vi "EnFlo_Lab_Temp_Control.vi"(0 "Current Time":dbl) -> ()   [LabVIEW 2016]
uses:
  <vilib>/Analysis/NI_AALPro.lvlib
panel:
  out "Integral Term":dbl
  out "Derivative Term":dbl
  out "Proportional Term":dbl
  out "Cooling from Tunnel Exit Duct kW":dbl
  out "Exit Heater Dem Power %":dbl
  in  "Ki":dbl=0.025 format="%.3f"
  in  "Kp":dbl=30.0 format="%.2f"
  in  "Kd":dbl=50.0 format="%.2f"
  in  "Derivative History":i32=20
  out "EnFlo_Tunnel:Temp:Pre_Inlet_Average":dbl
  out "EnFlo_Tunnel:Exit Duct:Dem Temp":dbl
  out "Reduction in air temp from ambient":dbl
  out "Heat Extraction Value in kW":dbl
  out "EnFlo Lab:Desired:Air Temp":dbl
  out "Temperature Error":dbl
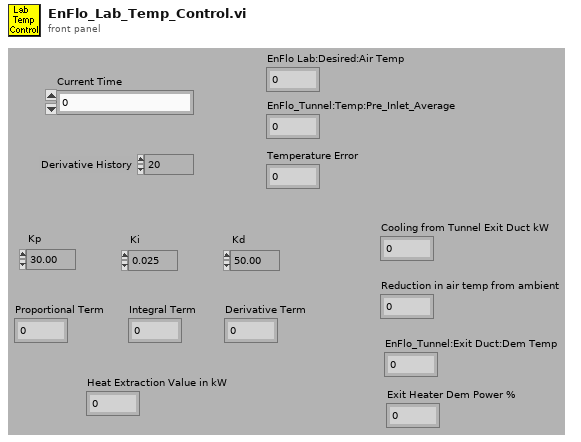
[diagram p1: front panel]
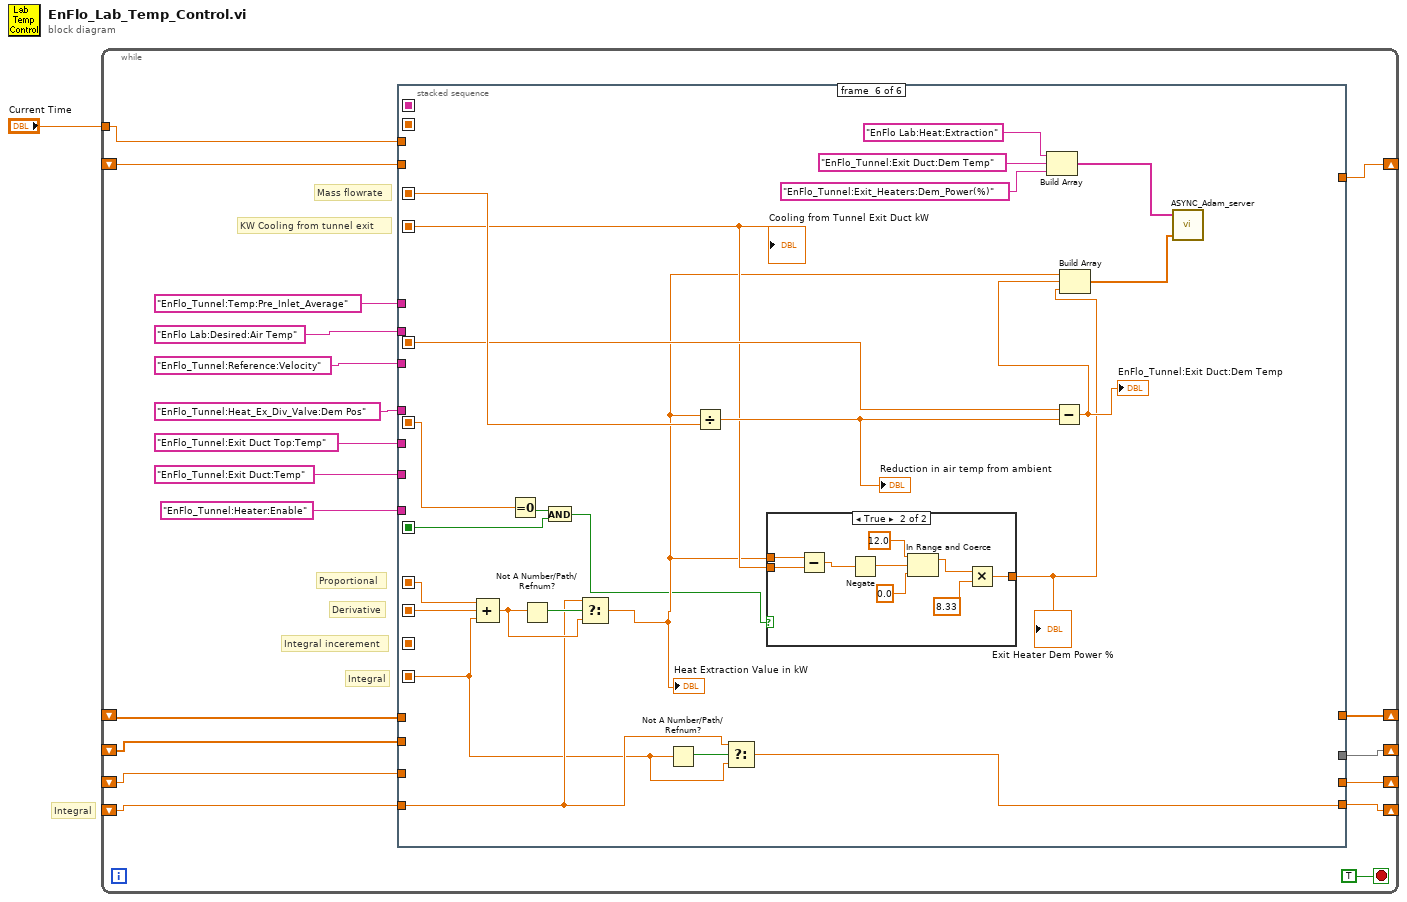
[diagram p0: block diagram]
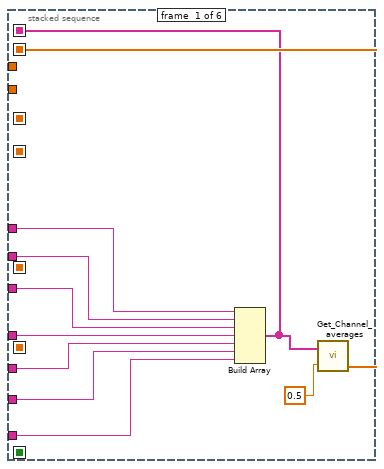
[diagram p2: hidden frame]
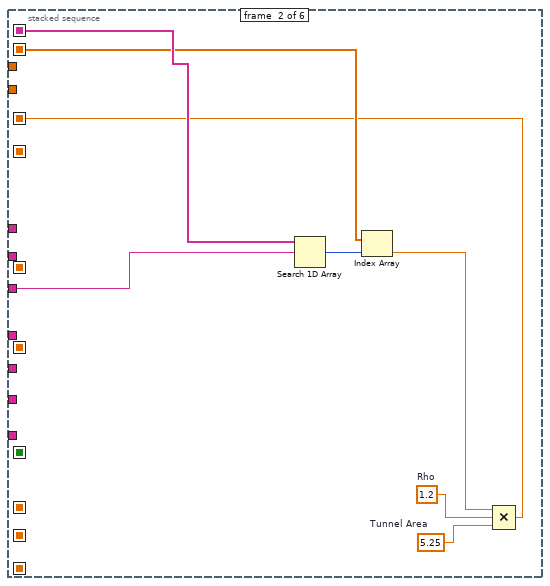
[diagram p3: hidden frame]
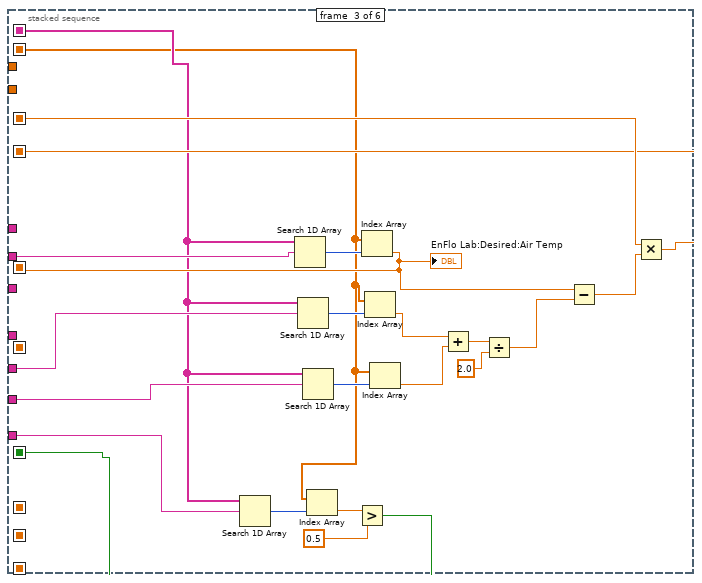
[diagram p4: hidden frame]
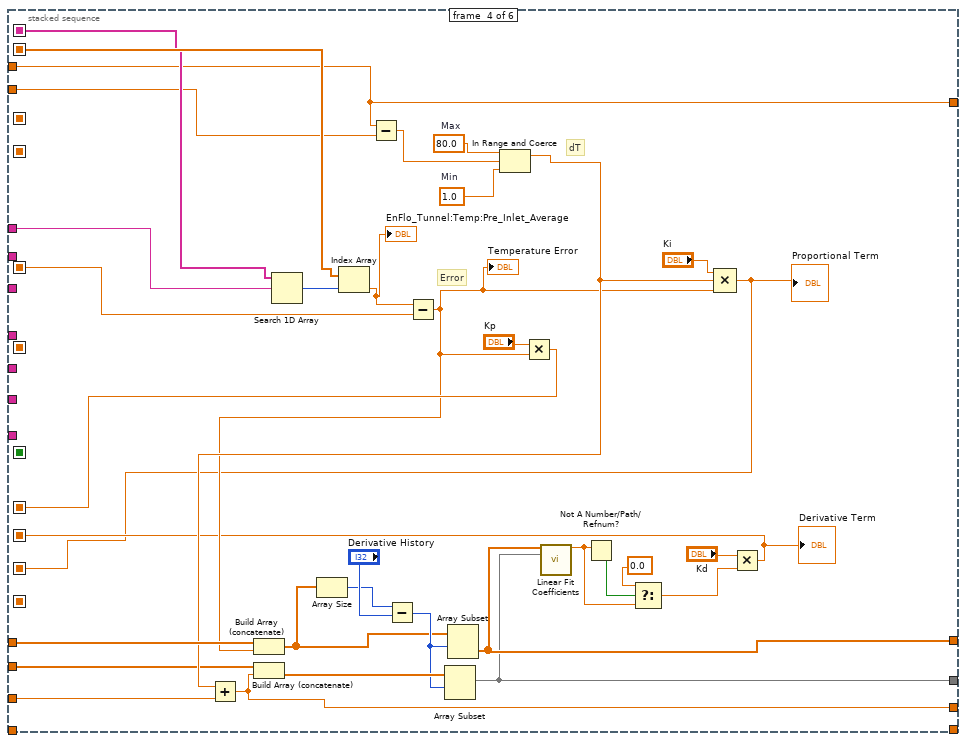
[diagram p5: hidden frame]
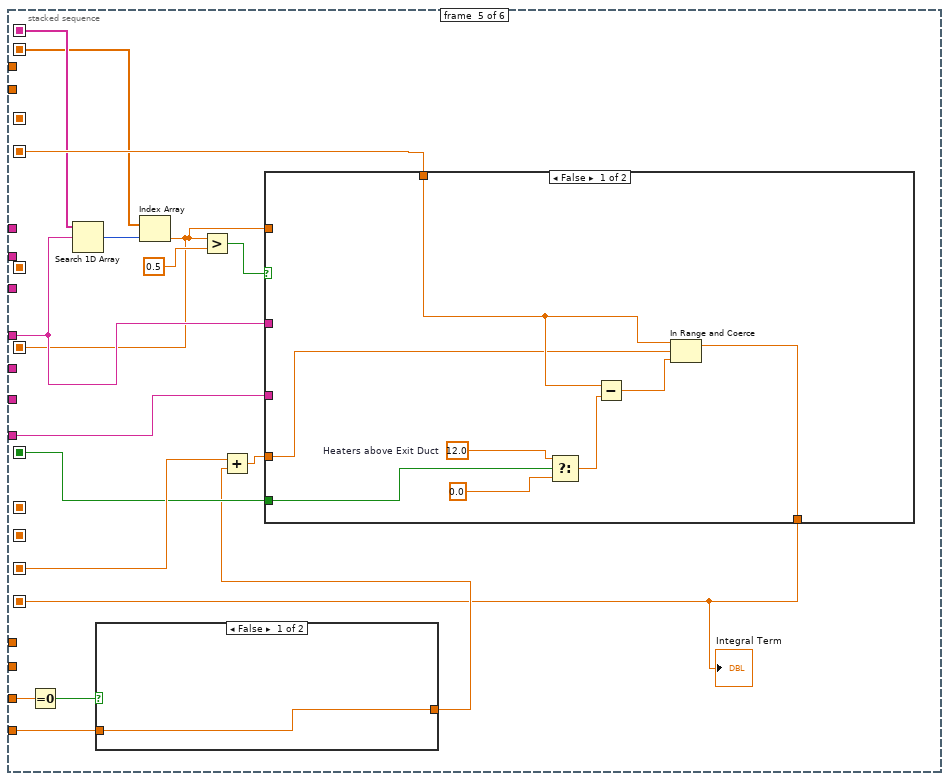
[diagram p6: hidden frame]
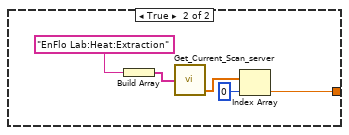
[diagram p7: hidden frame]
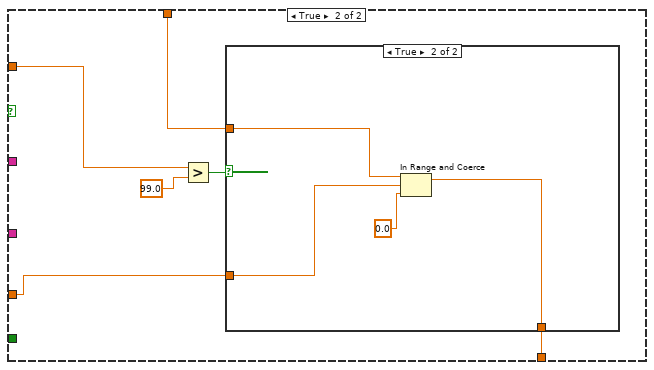
[diagram p8: hidden frame]
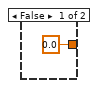
[diagram p10: hidden frame]
diagram:
  # "Integral"
  n1 = while {
    shift-right: [w8] -> _
    shift-left: _ -> [w9]
    shift-right: [w14] -> _
    shift-left: _ -> [w12]
    tunnel: "Current Time" -> [w13]
    shift-right: [w10] -> _
    shift-left: _ -> [w4]
    shift-right: [w11] -> _
    shift-left: _ -> [w7]
    shift-right: [w6] -> _
    shift-left: _ -> [w5]
    stop <- TRUE stop-if-true
    # "Integral"
    # "KW Cooling from tunnel exit"
    # "Mass flowrate"
    # "Integral incerement"
    # "Derivative"
    # "Proportional"
    n2 = stacked-sequence {
      seq-local: [w23 _ _ _ _ _] -> [_ w34 w41 w92 w103 _]
      seq-local: [w22 _ _ _ _ _] -> [_ w35 w42 w91 w104 _]
      seq-local: [_ _ _ w69 _ _] -> [_ _ _ _ _ w160]
      seq-local: [_ _ _ w62 _ _] -> [_ _ _ _ _ w159]
      seq-local: [_ _ _ w61 _ _] -> [_ _ _ _ w106 _]
      seq-local: [_ w31 _ _ _ _] -> [_ _ w48 _ _ w156]
      seq-local: [_ _ w47 _ _ _] -> [_ _ _ _ w107 w153]
      seq-local: [_ _ w46 _ _ _] -> [_ _ _ w66 _ w155]
      seq-local: [_ _ _ _ w95 _] -> [_ _ _ _ _ w143]
      seq-local: [_ _ w39 _ _ _] -> [_ _ _ _ w101 w138]
      seq-local: [_ _ _ _ w96 _] -> [_ _ _ _ _ w140]
      tunnel: "EnFlo_Tunnel:Temp:Pre_Inlet_Average" -> [w29 _ _ w93 _ _]
      tunnel: "EnFlo Lab:Desired:Air Temp" -> [w28 _ w57 _ _ _]
      tunnel: "EnFlo_Tunnel:Reference:Velocity" -> [w27 w33 _ _ _ _]
      tunnel: "EnFlo_Tunnel:Heat_Ex_Div_Valve:Dem Pos" -> [w26 _ _ _ w110 _]
      tunnel: "EnFlo_Tunnel:Exit Duct Top:Temp" -> [w25 _ w56 _ _ _]
      tunnel: "EnFlo_Tunnel:Exit Duct:Temp" -> [w24 _ w55 _ _ _]
      tunnel: [_ _ _ w90 _ _] -> w14
      tunnel: w13 -> [_ _ _ w90 _ _]
      tunnel: w12 -> [_ _ _ w89 _ _]
      tunnel: [_ _ _ w77 _ _] -> w11
      tunnel: [_ _ _ w76 _ _] -> w10
      tunnel: w9 -> [_ _ _ w75 w100 _]
      tunnel: [_ _ _ w74 _ _] -> w8
      tunnel: w7 -> [_ _ _ w73 _ _]
      tunnel: [_ _ _ _ _ w142] -> w6
      tunnel: w5 -> [_ _ _ _ w97 w144]
      tunnel: w4 -> [_ _ _ w63 _ _]
      tunnel: "EnFlo_Tunnel:Heater:Enable" -> [w21 _ w40 _ w102 _]
      frame #0 {
        n3 = Build Array(w29, w28, w27, w26, w25, w24, w21) -> (w22:string[])
        n4 = call "Get_Channel_averages.vi"("Desired Ch Names"=w22, "Averaging time (mins)"=0.5) -> ("number"=w23:dbl[])  [unwired: 1 in, 2 out]
      }
      frame #1 {
        w38 = 5.25  # Tunnel Area
        w37 = 1.2  # Rho
        n5 = Search 1D Array(1D array=w35, element=w33) -> (index of element=w36:i32)  [unwired: 1 out]
        n6 = Index Array(array=w34, index=w36) -> (element=w32:dbl)
        n7 = Compound Arithmetic op=MULTIPLY(w32, w37, w38) -> (w31:dbl)
      }
      frame #2 {
        n8 = Search 1D Array(1D array=w42, element=w40) -> (index of element=w45:i32)  [unwired: 1 out]
        n9 = Search 1D Array(1D array=w42, element=w57) -> (index of element=w60:i32)  [unwired: 1 out]
        n10 = Search 1D Array(1D array=w42, element=w56) -> (index of element=w59:i32)  [unwired: 1 out]
        n11 = Search 1D Array(1D array=w42, element=w55) -> (index of element=w58:i32)  [unwired: 1 out]
        n12 = Index Array(array=w41, index=w45) -> (element=w44:dbl)
        n13 = Greater?(x=w44, y=0.5) -> (0:w39:bool)
        n14 = Index Array(array=w41, index=w60) -> (element=w46:dbl)
        "EnFlo Lab:Desired:Air Temp" <- w46
        n15 = Index Array(array=w41, index=w59) -> (element=w54:dbl)
        n16 = Index Array(array=w41, index=w58) -> (element=w53:dbl)
        n17 = Add(x=w54, y=w53) -> (x+y=w52:dbl)
        n18 = Divide(x=w52, y=2.0) -> (x/y=w50:dbl)
        n19 = Subtract(x=w46, y=w50) -> (x-y=w49:dbl)
        n20 = Multiply(x=w48, y=w49) -> (x*y=w47:dbl)
      }
      frame #3 {
        w88 = 1.0  # Min
        w87 = 80.0  # Max
        # "dT"
        # "Error"
        n21 = Search 1D Array(1D array=w91, element=w93) -> (index of element=w94:i32)  [unwired: 1 out]
        n22 = Index Array(array=w92, index=w94) -> (element=w64:dbl)
        "EnFlo_Tunnel:Temp:Pre_Inlet_Average" <- w64
        n23 = Subtract(x=w90, y=w89) -> (x-y=w86:dbl)
        n24 = Subtract(x=w64, y=w66) -> (x-y=w65:dbl)
        "Temperature Error" <- w65
        n25 = Build Array (concatenate)(w73, w65) -> (w80:dbl[])
        n26 = Array Size(array=w80) -> (size(s)=w78:i32)
        n27 = Subtract(x=w78, y="Derivative History") -> (x-y=w81:i32)
        n28 = Array Subset(array=w80, index=w81) -> (w77:dbl[])  [unwired: 1 in]
        n29 = In Range and Coerce(upper limit=w87, x=w86, lower limit=w88) -> (coerced(x)=w68:dbl)  [unwired: 1 out]
        n30 = Add(x=w68, y=w75) -> (x+y=w74:dbl)
        n31 = Build Array (concatenate)(w63, w74) -> (w82:dbl[])
        n32 = Array Subset(array=w82, index=w81) -> (w76:dbl[])  [unwired: 1 in]
        n33 = Multiply(x="Kp", y=w65) -> (x*y=w69:dbl)
        n34 = call <vilib>:"Linear Fit Coefficients.vi"("Y"=w77, "X"=w76) -> ("slope"=w85:dbl)  [unwired: 3 in, 10 out]
        n35 = Not A Number/Path/Refnum?(number/path/refnum=w85) -> (NaN/Path/Refnum?=w83:bool)
        n36 = Select(t=0.0 ("f"), s=w83, f=w85) -> (s? t:f=w71:dbl)
        n37 = Compound Arithmetic op=MULTIPLY("Ki", w68, w65) -> (w61:dbl)
        "Proportional Term" <- w61
        n38 = Multiply(x="Kd", y=w71) -> (x*y=w62:dbl)
        "Derivative Term" <- w62
      }
      frame #4 {
        n39 = Equal To 0?(x=w100) -> (x = 0?=w99:bool)
        n40 = Search 1D Array(1D array=w104, element=w110) -> (index of element=w111:i32)  [unwired: 1 out]
        n41 = case shown="False" w99 {
          tunnel: [w112 w113] -> w98
          tunnel: w97 -> [w112 _]
          frame False {
          }
          frame True {
            n42 = Build Array("EnFlo Lab:Heat:Extraction") -> (w116:string[])
            n43 = call "Get_Current_Scan_server.vi"("Desired Channels"=w116) -> ("Numerical Values"=w115:dbl[])  [unwired: 2 out]
            n44 = Index Array(array=w115, index=0) -> (element=w113:dbl)
          }
        }
        n45 = Index Array(array=w103, index=w111) -> (element=w96:dbl)
        n46 = Greater?(x=w96, y=0.5) -> (0:w108:bool)
        n47 = Add(x=w106, y=w98) -> (x+y=w105:dbl)
        n48 = case shown="False" w108 {
          tunnel: w110 -> [_ _]
          tunnel: [w123 w129] -> w95
          tunnel: w96 -> [_ w128]
          tunnel: w107 -> [w125 w127]
          tunnel: w105 -> [w122 w126]
          tunnel: w102 -> [_ _]
          tunnel: w101 -> [w118 _]
          frame False {
            w121 = 12.0  # Heaters above Exit Duct
            n49 = Select(t=w121, s=w118, f=0.0) -> (s? t:f=w119:dbl)
            n50 = Subtract(x=w125, y=w119) -> (x-y=w124:dbl)
            n51 = In Range and Coerce(upper limit=w125, x=w122, lower limit=w124) -> (coerced(x)=w123:dbl)  [unwired: 1 out]
          }
          frame True {
            n52 = Greater?(x=w128, y=99.0) -> (0:w130:bool)
            n53 = case shown="True" w130 {
              tunnel: [w132 w133] -> w129
              tunnel: w127 -> [_ w136]
              tunnel: w126 -> [w132 w134]
              frame False {
              }
              frame True {
                n54 = In Range and Coerce(upper limit=w136, x=w134, lower limit=0.0) -> (coerced(x)=w133:dbl)  [unwired: 1 out]
              }
            }
          }
        }
        "Integral Term" <- w95
      }
      frame #5 {
        n55 = Compound Arithmetic op=ADD(w160, w159, w143) -> (w157:dbl)
        n56 = Equal To 0?(x=w140) -> (x = 0?=w139:bool)
        n57 = Not A Number/Path/Refnum?(number/path/refnum=w157) -> (NaN/Path/Refnum?=w158:bool)
        n58 = And(x=w139, y=w138) -> (x .and. y?=w137:bool)
        n59 = Select(t=w144, s=w158, f=w157) -> (s? t:f=w146:dbl)
        "Heat Extraction Value in kW" <- w146
        n60 = Not A Number/Path/Refnum?(number/path/refnum=w143) -> (NaN/Path/Refnum?=w145:bool)
        n61 = Divide(x=w146, y=w156) -> (x/y=w154:dbl)
        "Reduction in air temp from ambient" <- w154
        n62 = Select(t=w144, s=w145, f=w143) -> (s? t:f=w142:dbl)
        n63 = case shown="True" w137 {
          tunnel: w153 -> [_ w170]
          tunnel: [0.0 w163] -> w147
          tunnel: w146 -> [_ w162]
          frame False {
          }
          frame True {
            n64 = Subtract(x=w162, y=w170) -> (x-y=w164:dbl)
            n65 = Negate(x=w164) -> (-x=w165:dbl)
            n66 = In Range and Coerce(upper limit=12.0, x=w165, lower limit=0.0) -> (coerced(x)=w168:dbl)  [unwired: 1 out]
            n67 = Multiply(x=w168, y=8.33) -> (x*y=w163:dbl)
          }
        }
        "Exit Heater Dem Power %" <- w147
        n68 = Build Array("EnFlo Lab:Heat:Extraction", "EnFlo_Tunnel:Exit Duct:Dem Temp", "EnFlo_Tunnel:Exit_Heaters:Dem_Power(%)") -> (w149:string[])
        n69 = Subtract(x=w155, y=w154) -> (x-y=w148:dbl)
        "EnFlo_Tunnel:Exit Duct:Dem Temp" <- w148
        n70 = Build Array(w146, w148, w147) -> (w141:dbl[])
        n71 = call "ASYNC_Adam_server.vi"("Values"=w141, "Channel Names"=w149) -> ()  [unwired: 1 in, 3 out]
        "Cooling from Tunnel Exit Duct kW" <- w153
      }
    }
  }
